vi "MBus Connection Handle.vi"(8 "error in (no error)":errorcluster) -> (0 "error out":errorcluster)   [LabVIEW 2018]
uses:
  CTL/FGV - R-W.ctl
  <vilib>/NI/Modbus Library/API/Wrapper/Create Serial Master.vi
  <vilib>/NI/Modbus Library/API/master/Modbus Master.lvclass
  <vilib>/NI/Modbus Library/API/Wrapper/API Main.lvlib
panel:
  out "dt":u32
  out "loop error":errorcluster
  out "MBus Data":bool[](array[boolean])
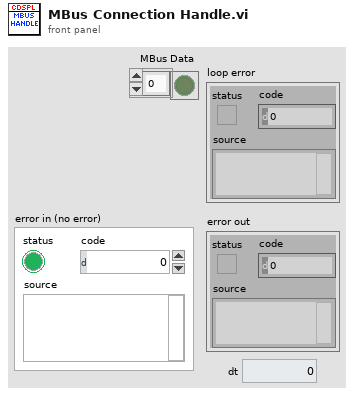
[diagram p1: front panel]
types:
  T1 = typedef "FGV - R-W.ctl" = enum16{"W", "R"}
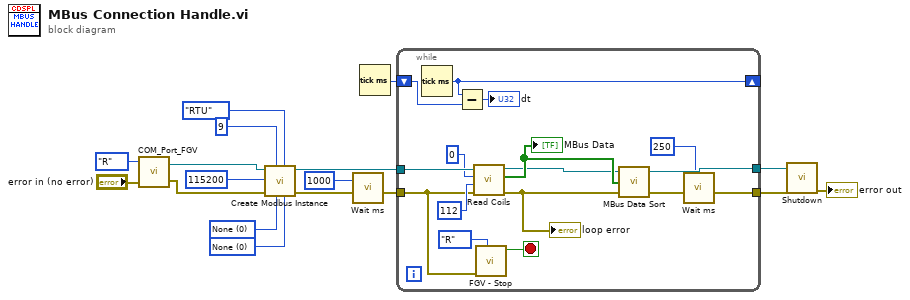
[diagram p0: block diagram]
diagram:
  w15 = u16 0 items=["None", "XON/XOFF", "RTS/CTS", "XON/XOFF & RTS/CTS", "DTR/DSR", "XON/XOFF & DTR/DSR"] ("flow control (none)")
  w16 = u16 0 items=["None", "Odd", "Even", "Mark", "Space"] ("parity (even)")
  n1 = call "COM_Port_FGV.vi"("error in (no error)"="error in (no error)", "Action"=FGV_-_R-W."R") -> ("error out"=w2:errorcluster, "COM Port Out"=w3:refnum<visa-resource-name>)  [unwired: 1 in]
  n2 = call-poly <vilib>:"Create Modbus Instance.vi"("flow control (none)"=w15, "serial type"=enum16{"RTU", "ASCII"}."RTU", "parity (even)"=w16, "unit ID"=u8 9, "error in"=w2, "baud rate"=u32 115200, "VISA resource name"=w3) -> ("error out"=w8:errorcluster, "serial master instance"=w12:refnum<class "Modbus Master.lvclass">)  [unwired: 3 in]
  n3 = call "Wait ms.vi"("milliseconds to wait"=u32 1000, "error in (no error)"=w8) -> ("error out"=w7:errorcluster)  [unwired: 9 in]
  n4 = Tick Count (ms)() -> (millisecond timer value=w5:u32)
  n5 = while {
    tunnel: w12 -> [w33]
    tunnel: w7 -> [w27]
    tunnel: [w19] -> w11
    tunnel: [w22] -> w10
    shift-right: [w28] -> _
    shift-left: w5 -> [w29]
    stop <- w25 stop-if-true
    n6 = Tick Count (ms)() -> (millisecond timer value=w28:u32)
    n7 = Subtract(x=w28, y=w29) -> (x-y=→"dt":u32)
    n8 = call-dynamic "Read Coils.vi"("error in"=w27, "number of inputs"=u16 112, "starting address"=u16 0, "Modbus master in"=w33) -> ("error out"=w21:errorcluster, "coils"=w24:bool[], "Modbus master out"=w23:refnum<class "Modbus Master.lvclass">)  [unwired: 5 in]
    "MBus Data" <- w24
    "loop error" <- w21
    n9 = call "FGV - Stop.vi"("Action"=FGV_-_R-W."R", "error in (no error)"=w27) -> ("Acquire? Out"=w25:bool)  [unwired: 8 in, 1 out]
    n10 = call "MBus Data Sort.vi"("Error In"=w21, "Raw Input Data"=w24, "Modbus master in"=w23) -> ("Error Out"=w20:errorcluster, "Modbus master out"=w22:refnum<class "Modbus Master.lvclass">)  [unwired: 1 out]
    n11 = call "Wait ms.vi"("milliseconds to wait"=u32 250, "error in (no error)"=w20) -> ("error out"=w19:errorcluster)  [unwired: 9 in]
  }
  n12 = call-dynamic "Shutdown.vi"("error in"=w11, "Modbus master in"=w10) -> ("error out"=→"error out":errorcluster)  [unwired: 9 in]
